vi "parse-rack.vi"(1 "reading":cluster{"address":u16, "value":u16}[](array[cluster])) -> (0 "rack":T1)   [LabVIEW 2021]
uses:
  General Purpose/BMS.ctl
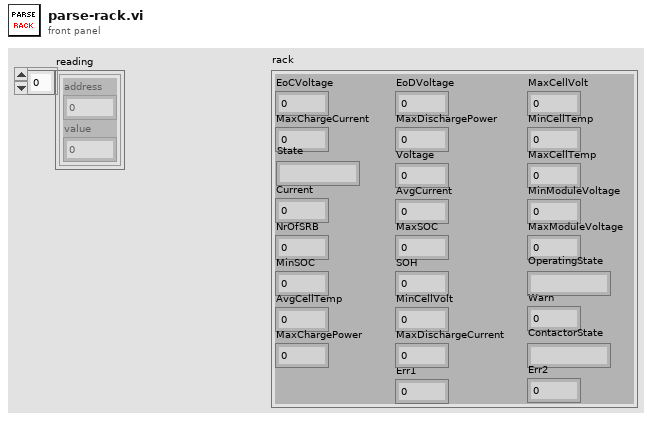
[diagram p1: front panel]
types:
  T1 = cluster{"EoCVoltage":dbl, "MaxChargeCurrent":dbl, "EoDVoltage":dbl, "MaxDischargePower":dbl, "Voltage":dbl, "Current":dbl, "NrOfSRB":u16, "AvgCurrent":dbl, "MaxSOC":u16, "MinSOC":u16, "MaxCellVolt":dbl, "MinCellTemp":dbl, "SOH":u16, "MaxCellTemp":dbl, "AvgCellTemp":dbl, "MinCellVolt":dbl, "MinModuleVoltage":dbl, "MaxModuleVoltage":dbl, "Err1":u16, "Warn":u16, "MaxChargePower":dbl, "MaxDischargeCurrent":dbl, "State":string, "ContactorState":string, "OperatingState":string, "Err2":u16}
  T2 = typedef "BMS.ctl" = cluster{"rack":cluster{"EoCVoltage":dbl, "MaxChargeCurrent":dbl, "EoDVoltage":dbl, "MaxDischargePower":dbl, "Voltage":dbl, "Current":dbl, "NrOfSRB":u16, "AvgCurrent":dbl, "MaxSOC":u16, "MinSOC":u16, "MaxCellVolt":dbl, "MinCellTemp":dbl, "SOH":u16, "MaxCellTemp":dbl, "AvgCellTemp":dbl, "MinCellVolt":dbl, "MinModVoltage":dbl, "MaxModVoltage":dbl, "Err1":u16, "Warn":u16, "MaxChargePower":dbl, "MaxDischargeCurrent":dbl, "State":string, "ContactorState":string, "OperatingState":string, "Err2":u16}[], "modules":cluster{"Voltage":dbl, "MaxCellTemp":dbl, "AirTempIn":dbl, "MinCellVoltage":u16, "AirTempOut":dbl, "MinSOC":u16, "MaxCellVoltage":u16, "Warn":u16, "SOH":u16, "MinCellTemp":dbl, "Err":u16, "Max SOC":u16}[]}
  T3 = cluster{"EoCVoltage":dbl, "MaxChargeCurrent":dbl, "EoDVoltage":dbl, "MaxDischargePower":dbl, "Voltage":dbl, "Current":dbl, "NrOfSRB":u16, "AvgCurrent":dbl, "MaxSOC":u16, "MinSOC":u16, "MaxCellVolt":dbl, "MinCellTemp":dbl, "SOH":u16, "MaxCellTemp":dbl, "AvgCellTemp":dbl, "MinCellVolt":dbl, "MinModVoltage":dbl, "MaxModVoltage":dbl, "Err1":u16, "Warn":u16, "MaxChargePower":dbl, "MaxDischargeCurrent":dbl, "State":string, "ContactorState":string, "OperatingState":string, "Err2":u16}[]
  T4 = cluster{"EoCVoltage":dbl, "MaxChargeCurrent":dbl, "EoDVoltage":dbl, "MaxDischargePower":dbl, "Voltage":dbl, "Current":dbl, "NrOfSRB":u16, "AvgCurrent":dbl, "MaxSOC":u16, "MinSOC":u16, "MaxCellVolt":dbl, "MinCellTemp":dbl, "SOH":u16, "MaxCellTemp":dbl, "AvgCellTemp":dbl, "MinCellVolt":dbl, "MinModVoltage":dbl, "MaxModVoltage":dbl, "Err1":u16, "Warn":u16, "MaxChargePower":dbl, "MaxDischargeCurrent":dbl, "State":string, "ContactorState":string, "OperatingState":string, "Err2":u16}
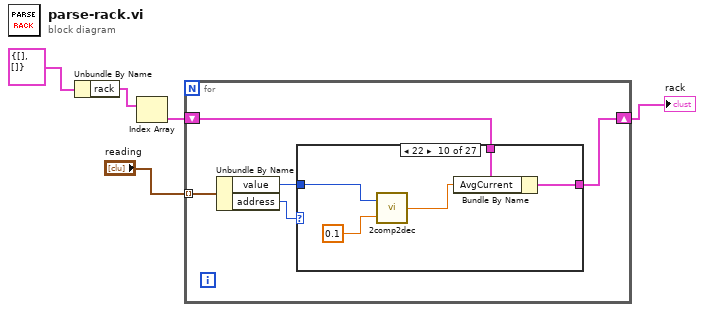
[diagram p0: block diagram]
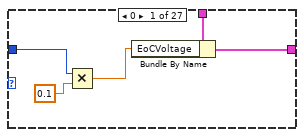
[diagram p2: hidden frame]
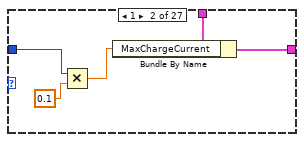
[diagram p3: hidden frame]
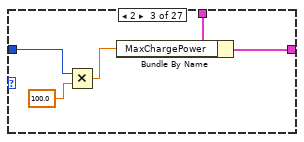
[diagram p4: hidden frame]
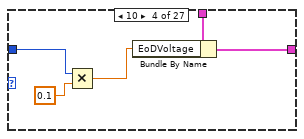
[diagram p5: hidden frame]
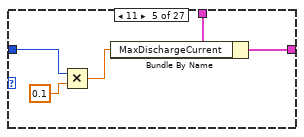
[diagram p6: hidden frame]
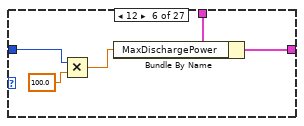
[diagram p7: hidden frame]
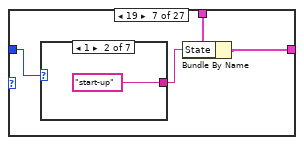
[diagram p8: hidden frame]
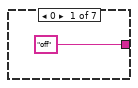
[diagram p9: hidden frame]
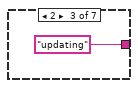
[diagram p10: hidden frame]
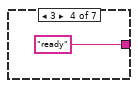
[diagram p11: hidden frame]
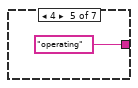
[diagram p12: hidden frame]
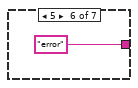
[diagram p13: hidden frame]
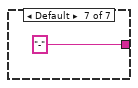
[diagram p14: hidden frame]
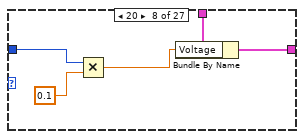
[diagram p15: hidden frame]
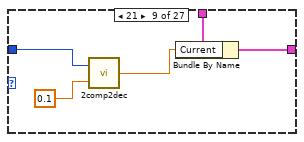
[diagram p16: hidden frame]
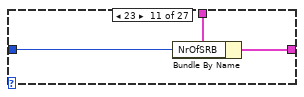
[diagram p17: hidden frame]
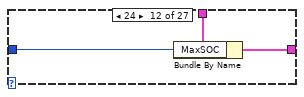
[diagram p18: hidden frame]
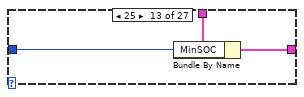
[diagram p19: hidden frame]
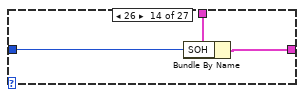
[diagram p20: hidden frame]
diagram:
  n1 = Unbundle By Name(T2 {"rack"=[], "modules"=[]} ("BMS")) -> ("rack"=w3:T3)
  n2 = Index Array(array=w3) -> (element=w2:T4)  [unwired: 1 in]
  n3 = for {
    tunnel: "reading" -> [w10] mode=indexing
    shift-right: [w6] -> w1
    shift-left: w2 -> [w7]
    n4 = Unbundle By Name(w10) -> ("value"=w8:u16, "address"=w9:u16)
    n5 = case shown="22" w9 {
      tunnel: w8 -> [w13 w18 w22 w28 w33 w37 w42 w53 w59 w63 w67 w70 w73 w76 w80 w85 w93 w98 w103 w107 w110 w115 w121 w128 w131 w134 _]
      tunnel: w7 -> [w15 w20 w25 w30 w35 w40 w44 w56 w61 w66 w69 w72 w75 w78 w83 w87 w96 w101 w105 w109 w114 w119 w123 w130 w133 w136 w137]
      tunnel: [w14 w19 w24 w29 w34 w39 w43 w55 w60 w65 w68 w71 w74 w77 w82 w86 w95 w100 w104 w108 w113 w118 w122 w129 w132 w135 w137] -> w6
      frame 0 {
        n6 = Multiply(x=w13, y=0.1) -> (x*y=w12:dbl)
        n7 = Bundle By Name(cluster=w15, "EoCVoltage"=w12) -> (w14:T4)
      }
      frame 1 {
        n8 = Multiply(x=w18, y=0.1) -> (x*y=w16:dbl)
        n9 = Bundle By Name(cluster=w20, "MaxChargeCurrent"=w16) -> (w19:T4)
      }
      frame 2 {
        n10 = Multiply(x=w22, y=100.0) -> (x*y=w21:dbl)
        n11 = Bundle By Name(cluster=w25, "MaxChargePower"=w21) -> (w24:T4)
      }
      frame 10 {
        n12 = Multiply(x=w28, y=0.1 ("x")) -> (x*y=w26:dbl)
        n13 = Bundle By Name(cluster=w30, "EoDVoltage"=w26) -> (w29:T4)
      }
      frame 11 {
        n14 = Multiply(x=w33, y=0.1) -> (x*y=w31:dbl)
        n15 = Bundle By Name(cluster=w35, "MaxDischargeCurrent"=w31) -> (w34:T4)
      }
      frame 12 {
        n16 = Multiply(x=w37, y=100.0) -> (x*y=w36:dbl)
        n17 = Bundle By Name(cluster=w40, "MaxDischargePower"=w36) -> (w39:T4)
      }
      frame 19 {
        n18 = case shown="1" w42 {
          tunnel: ["off" "start-up" "updating" "ready" "operating" "error" "-"] -> w41
          frame 0 {
          }
          frame 1 {
          }
          frame 2 {
          }
          frame 3 {
          }
          frame 4 {
          }
          frame 5 {
          }
          frame Default {
          }
        }
        n19 = Bundle By Name(cluster=w44, "State"=w41) -> (w43:T4)
      }
      frame 20 {
        n20 = Multiply(x=w53, y=0.1) -> (x*y=w52:dbl)
        n21 = Bundle By Name(cluster=w56, "Voltage"=w52) -> (w55:T4)
      }
      frame 21 {
        n22 = call "2comp2dec.vi"("factor"=0.1, "two' complement"=w59) -> ("decimal"=w58:dbl)  [unwired: 1 in]
        n23 = Bundle By Name(cluster=w61, "Current"=w58) -> (w60:T4)
      }
      frame 22 {
        n24 = call "2comp2dec.vi"("factor"=0.1, "two' complement"=w63) -> ("decimal"=w62:dbl)  [unwired: 1 in]
        n25 = Bundle By Name(cluster=w66, "AvgCurrent"=w62) -> (w65:T4)
      }
      frame 23 {
        n26 = Bundle By Name(cluster=w69, "NrOfSRB"=w67) -> (w68:T4)
      }
      frame 24 {
        n27 = Bundle By Name(cluster=w72, "MaxSOC"=w70) -> (w71:T4)
      }
      frame 25 {
        n28 = Bundle By Name(cluster=w75, "MinSOC"=w73) -> (w74:T4)
      }
      frame 26 {
        n29 = Bundle By Name(cluster=w78, "SOH"=w76) -> (w77:T4)
      }
      frame 31 {
        n30 = call "2comp2dec.vi"("factor"=1.0, "two' complement"=w80) -> ("decimal"=w79:dbl)  [unwired: 1 in]
        n31 = Bundle By Name(cluster=w83, "AvgCellTemp"=w79) -> (w82:T4)
      }
      frame 33 {
        n32 = case shown="2" w85 {
          tunnel: ["open" "pre-charge" "closed" "-"] -> w84
          frame 0 {
          }
          frame 1 {
          }
          frame 2 {
          }
          frame Default {
          }
        }
        n33 = Bundle By Name(cluster=w87, "ContactorState"=w84) -> (w86:T4)
      }
      frame 34 {
        n34 = Multiply(x=w93, y=0.001) -> (x*y=w92:dbl)
        n35 = Bundle By Name(cluster=w96, "MinCellVolt"=w92) -> (w95:T4)
      }
      frame 35 {
        n36 = Multiply(x=w98, y=0.001) -> (x*y=w97:dbl)
        n37 = Bundle By Name(cluster=w101, "MaxCellVolt"=w97) -> (w100:T4)
      }
      frame 36 {
        n38 = call "2comp2dec.vi"("two' complement"=w103) -> ("decimal"=w102:dbl)  [unwired: 2 in]
        n39 = Bundle By Name(cluster=w105, "MinCellTemp"=w102) -> (w104:T4)
      }
      frame 37 {
        n40 = call "2comp2dec.vi"("two' complement"=w107) -> ("decimal"=w106:dbl)  [unwired: 2 in]
        n41 = Bundle By Name(cluster=w109, "MaxCellTemp"=w106) -> (w108:T4)
      }
      frame 38 {
        n42 = Multiply(x=w110, y=0.01) -> (x*y=w112:dbl)
        n43 = Bundle By Name(cluster=w114, "MinModVoltage"=w112) -> (w113:T4)
      }
      frame 39 {
        n44 = Multiply(x=w115, y=0.01) -> (x*y=w117:dbl)
        n45 = Bundle By Name(cluster=w119, "MaxModVoltage"=w117) -> (w118:T4)
      }
      frame 52 {
        n46 = case shown="Default" w121 {
          tunnel: ["discharge" "charge" "idle" "-"] -> w120
          frame 1 {
          }
          frame 2 {
          }
          frame 3 {
          }
          frame Default {
          }
        }
        n47 = Bundle By Name(cluster=w123, "OperatingState"=w120) -> (w122:T4)
      }
      frame 70 {
        n48 = Bundle By Name(cluster=w130, "Err1"=w128) -> (w129:T4)
      }
      frame 71 {
        n49 = Bundle By Name(cluster=w133, "Err2"=w131) -> (w132:T4)
      }
      frame 74 {
        n50 = Bundle By Name(cluster=w136, "Warn"=w134) -> (w135:T4)
      }
      frame Default {
      }
    }
  }
  "rack" <- w1
